vi "TcA03-007_TimeoutWhenWaitingForModifyingClassAttributes.vi"(1 "Input buffer":T3="1", 3 "Invocation info":T2, 5 "error in (no error)":errorcluster, 6 "Add log to result?":bool) -> (16 "Test Data":T1 {"Numeric Measurement" format="%.2f"}, 19 "error out":errorcluster)   [LabVIEW 2020]
doc: "Test case template."
uses:
  Shared/Support_InputBuffer.ctl
  Shared/Support_InvocationInfo.ctl
  Shared/Support_TestData.ctl
  <vilib>/addons/_AddQ/G#Object/G#Object.lvclass
  TestClasses/G#SubClass2_class/G#SubClass2.lvclass
  TestClasses/G#BaseClass2_class/G#BaseClass2.lvclass
panel:
  in  "Test name":string="TcA03-007 Timeout when waiting for modifying class attributes"
  out "Test result":bool
  out "Result":string
  # "Verify that waiting for modifying class attributes\nwhen mutual excluded can be timeout."
  # "Sub test case"
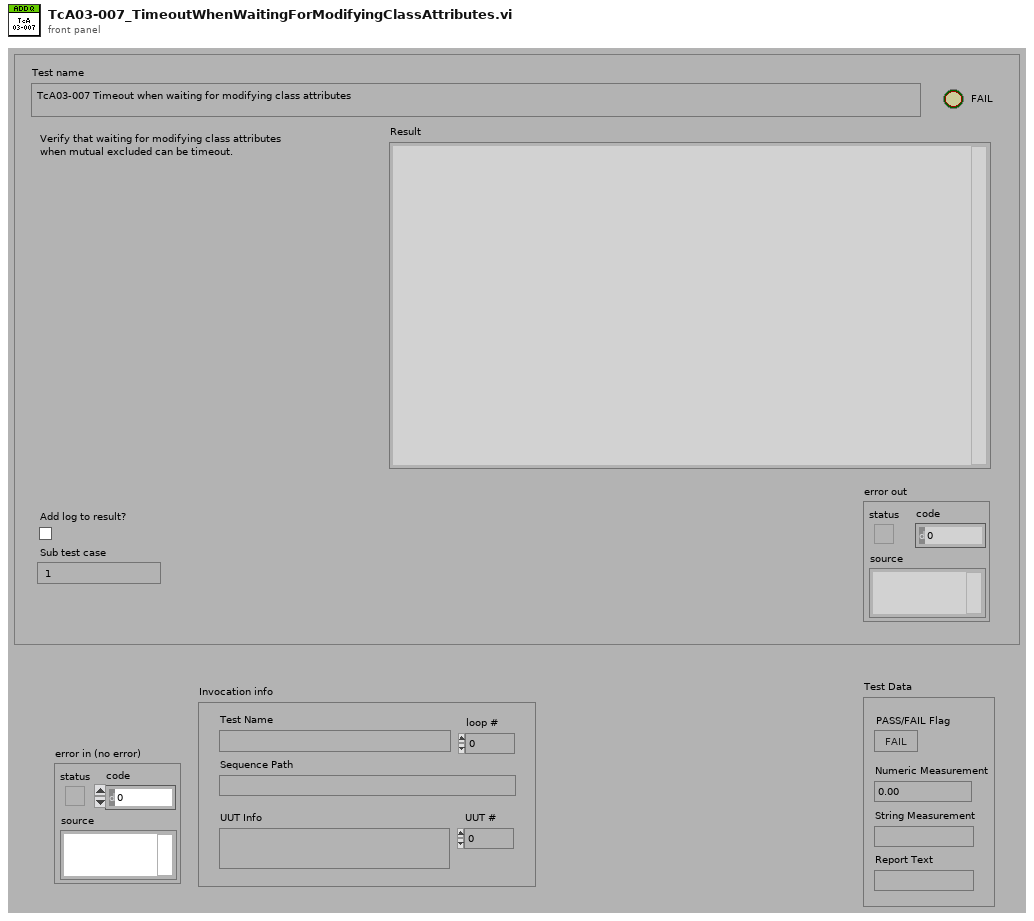
[diagram p1: front panel]
types:
  T1 = typedef "Support_TestData.ctl" = cluster{"PASS/FAIL Flag":bool, "Numeric Measurement":dbl, "String Measurement":string, "Report Text":string}
  T2 = typedef "Support_InvocationInfo.ctl" = cluster{"UUT #":i32, "loop #":i32, "UUT Info":string, "Test Name":string, "Sequence Path":path}
  T3 = typedef "Support_InputBuffer.ctl" = string
  T4 = typedef "Support_ResultType.ctl" = cluster{"Pass":bool, "Comment":string, "MeasurementValue":dbl}
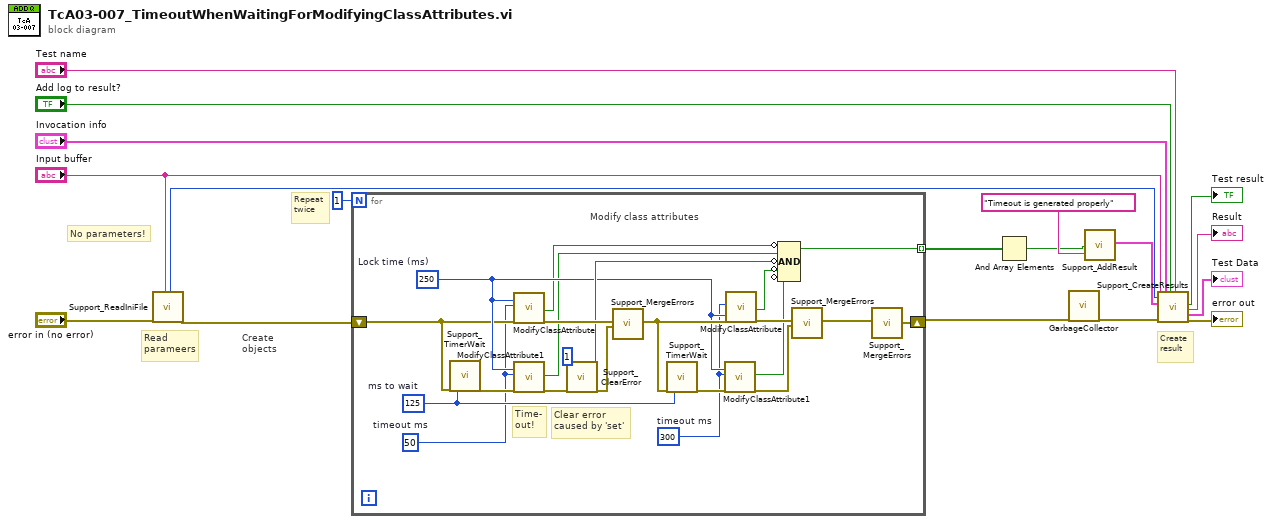
[diagram p0: block diagram]
diagram:
  # "Repeat\ntwice"
  # "Create\nobjects"
  # "No parameters!"
  # "Create\nresult"
  # "Read\nparameers"
  n1 = call "Support_ReadIniFile.vi"("error in (no error)"="error in (no error)", "Sub test case"="Input buffer") -> ("Timer start"=w9:u32, "error out"=w2:errorcluster)  [unwired: 10 in, 6 out]
  n2 = for {
    N: 1 -> [_]
    tunnel: [w24] -> w5 mode=indexing
    shift-right: [w27] -> w1
    shift-left: w2 -> [w26]
    w25 = 300  # timeout ms
    w23 = 50  # timeout ms
    w29 = u32 250  # Lock time (ms)
    w28 = u32 125  # ms to wait
    # "Time-\nout!"
    # "Clear error\ncaused by 'set'"
    # "Modify class attributes"
    n3 = call "Support_TimerWait.vi"("error in (no error)"=w26, "milliseconds to wait"=w28) -> ("error out"=w39:errorcluster)  [unwired: 17 in]
    n4 = call "ModifyClassAttribute.vi"("Lock time (ms)"=w29, "timeout in ms (-1)"=w23, "error in (no error)"=w26) -> ("timeout"=w22:bool, "error out"=w40:errorcluster)  [unwired: 14 in, 1 out]
    n5 = call "ModifyClassAttribute1.vi"("Lock time (ms)"=w29, "timeout in ms (-1)"=w23, "error in (no error)"=w39) -> ("timeout"=w21:bool, "error out"=w33:errorcluster)  [unwired: 14 in, 1 out]
    n6 = call "Support_ClearError.vi"("code"=1, "error in (no error)"=w33) -> ("Cleared?"=w30:bool, "error out"=w32:errorcluster)  [unwired: 16 in]
    n7 = call "Support_MergeErrors.vi"("error in 1"=w40, "error in 2"=w32) -> ("error out"=w34:errorcluster)  [unwired: 16 in, 1 out]
    n8 = call "Support_TimerWait.vi"("error in (no error)"=w34, "milliseconds to wait"=w28) -> ("error out"=w36:errorcluster)  [unwired: 17 in]
    n9 = call "ModifyClassAttribute1.vi"("Lock time (ms)"=w29, "timeout in ms (-1)"=w25, "error in (no error)"=w36) -> ("timeout"=w19:bool, "error out"=w37:errorcluster)  [unwired: 14 in, 1 out]
    n10 = call "ModifyClassAttribute.vi"("Lock time (ms)"=w29, "timeout in ms (-1)"=w25, "error in (no error)"=w34) -> ("timeout"=w20:bool, "error out"=w38:errorcluster)  [unwired: 14 in, 1 out]
    n11 = Compound Arithmetic op=AND(invert w22, w21, invert w30, invert w20, invert w19) -> (w24:bool)
    n12 = call "Support_MergeErrors.vi"("error in 1"=w38, "error in 2"=w37) -> ("error out"=w35:errorcluster)  [unwired: 16 in, 1 out]
    n13 = call "Support_MergeErrors.vi"("error in 1"=w35) -> ("error out"=w27:errorcluster)  [unwired: 17 in, 1 out]
  }
  n14 = And Array Elements(Boolean array=w5) -> (logical AND=w4:bool)
  n15 = call <vilib>:"GarbageCollector.vi"("error in (no error)"=w1) -> ("error out"=w8:errorcluster)  [unwired: 16 in, 2 out]
  n16 = call "Support_AddResult.vi"("Pass"=w4, "Comment"="Timeout is generated properly") -> ("Results out"=w7:T4[])  [unwired: 17 in]
  n17 = call "Support_CreateResults.vi"("Sub test case"="Input buffer", "Timer start"=w9, "Results"=w7, "error in (no error)"=w8, "Invocation info"="Invocation info", "Add log to result?"="Add log to result?", "Test name"="Test name") -> ("Pass/fail flag"=→"Test result":bool, "Result"=→"Result":string, "Test Data"=→"Test Data":T1, "error out"=→"error out":errorcluster)  [unwired: 9 in]
